vi "canmotor.vi"() -> (0 "x < y?":bool, 1 "两路电机速度":string, 2 "J45电机":dbl, 3 "J67电机":dbl)   [LabVIEW 2020]
uses:
  ControlCAN For LabVIEW8.6/ControlCAN.llb/VCI_CAN_OBJ.ctl
  ControlCAN For LabVIEW8.6/ControlCAN.llb/DevType.ctl
  ControlCAN For LabVIEW8.6/ControlCAN.llb/VCI_INIT_CONFIG.ctl
  ControlCAN For LabVIEW8.6/ControlCAN.llb/InitFlag.ctl
  ControlCAN For LabVIEW8.6/ControlCAN.llb/Fliter.ctl
  ControlCAN For LabVIEW8.6/ControlCAN.llb/Mode.ctl
  ControlCAN For LabVIEW8.6/ControlCAN.lvlib
panel:
  out "十进制整型字符串 2":string
  out "十进制整型字符串":string
  out "输出结果－电子表格字符串（'\\'代码显示） 2":string
  out "电机和":dbl
  out "Recieve 2":T1[](array[typedef])
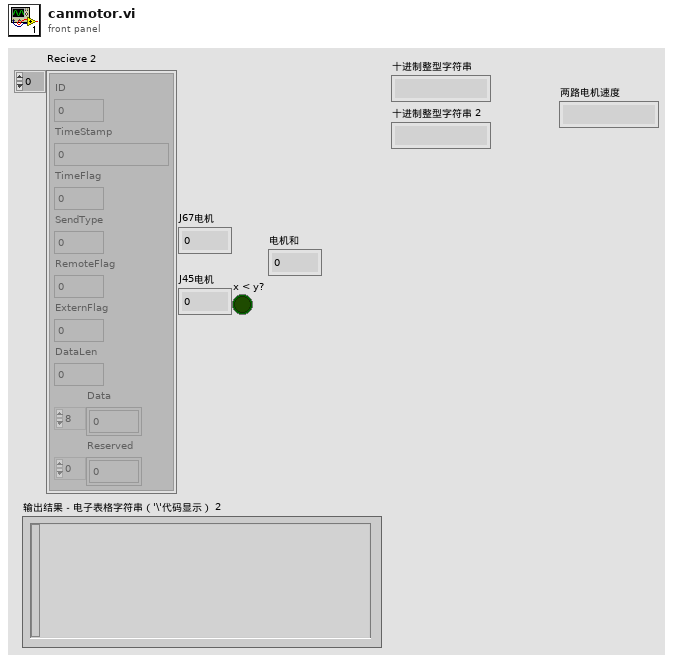
[diagram p1: front panel]
types:
  T1 = typedef "ControlCAN.lvlib/VCI_CAN_OBJ.ctl" = cluster{"ID":u32, "TimeStamp":u32, "TimeFlag":u8, "SendType":u8, "RemoteFlag":u8, "ExternFlag":u8, "DataLen":u8, "Data":u8[], "Reserved":u8[]}
  T2 = typedef "ControlCAN.lvlib/VCI_INIT_CONFIG.ctl" = cluster{"AccCode":u32, "AccMask":u32, "InitFlag":T3, "Fliter":T4, "Timing0":u8, "Timing1":u8, "Mode":T5}
  T3 = typedef "ControlCAN.lvlib/InitFlag.ctl" = u32
  T4 = typedef "ControlCAN.lvlib/Fliter.ctl" = u8
  T5 = typedef "ControlCAN.lvlib/Mode.ctl" = u8
  T6 = typedef "ControlCAN.lvlib/DevType.ctl" = u32
  T7 = cluster{"Recieve 2[0]":T1, "Recieve 2[1]":T1, "Recieve 2[2]":T1, "Recieve 2[3]":T1, "Recieve 2[4]":T1, "Recieve 2[5]":T1, "Recieve 2[6]":T1, "Recieve 2[7]":T1, "Recieve 2[8]":T1}
  T8 = cluster{"Data[0]":u8, "Data[1]":u8, "Data[2]":u8, "Data[3]":u8, "Data[4]":u8, "Data[5]":u8, "Data[6]":u8, "Data[7]":u8, "Data[8]":u8}
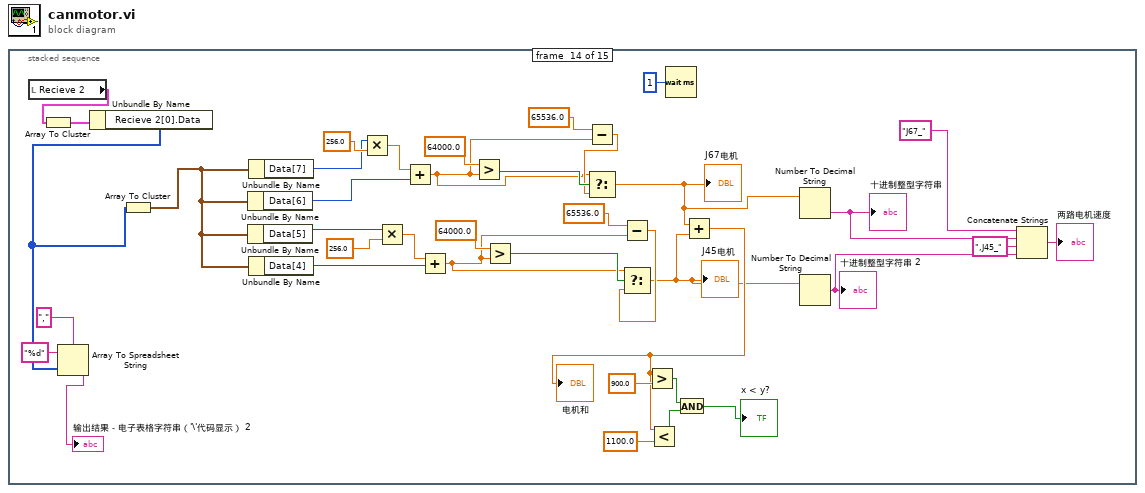
[diagram p0: block diagram]
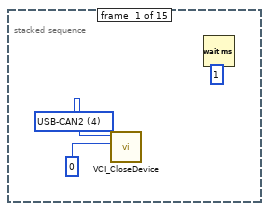
[diagram p2: hidden frame]
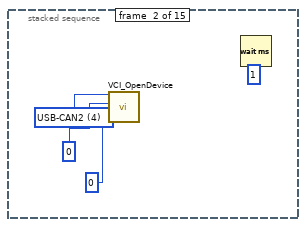
[diagram p3: hidden frame]
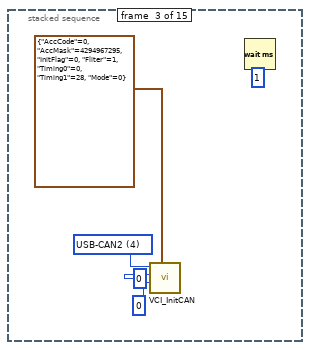
[diagram p4: hidden frame]
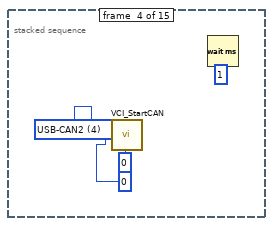
[diagram p5: hidden frame]
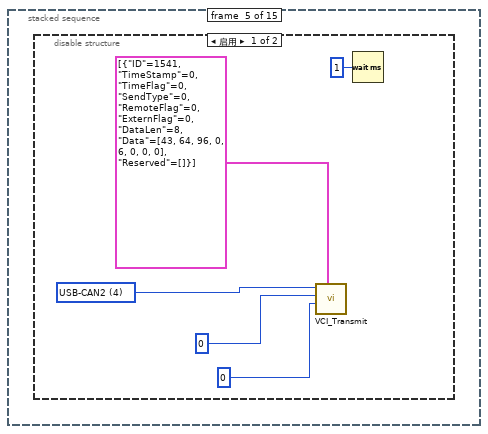
[diagram p6: hidden frame]
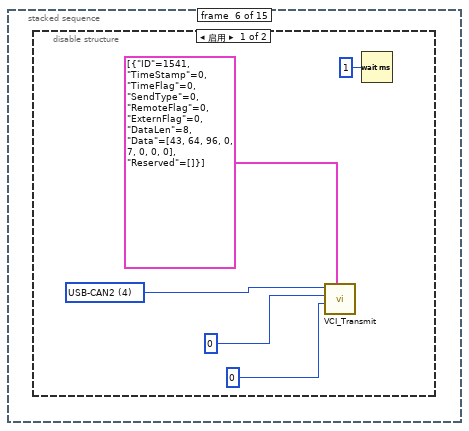
[diagram p8: hidden frame]
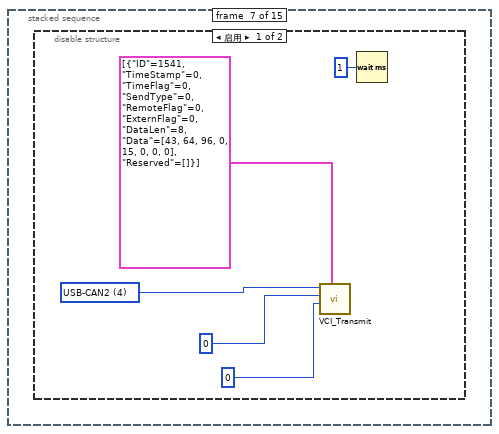
[diagram p10: hidden frame]
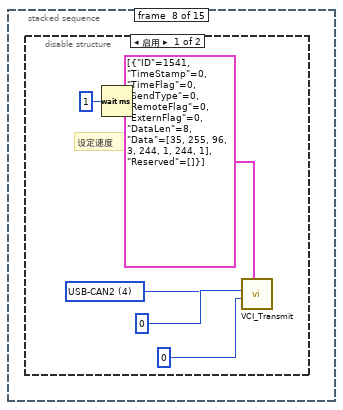
[diagram p12: hidden frame]
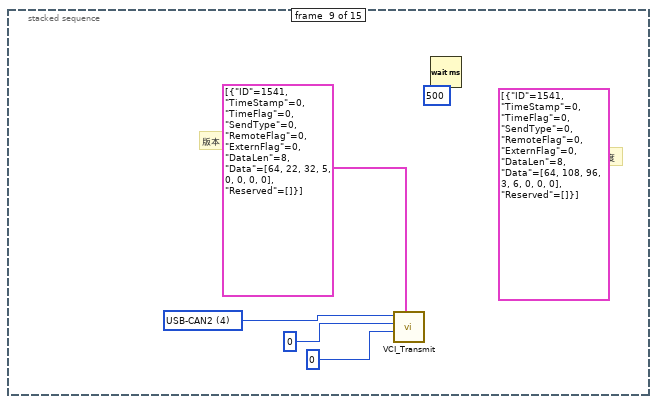
[diagram p14: hidden frame]
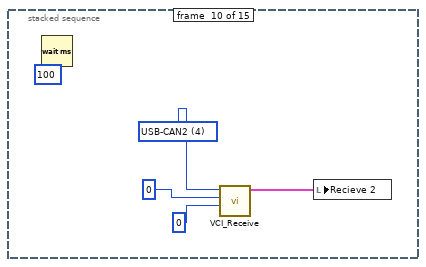
[diagram p15: hidden frame]
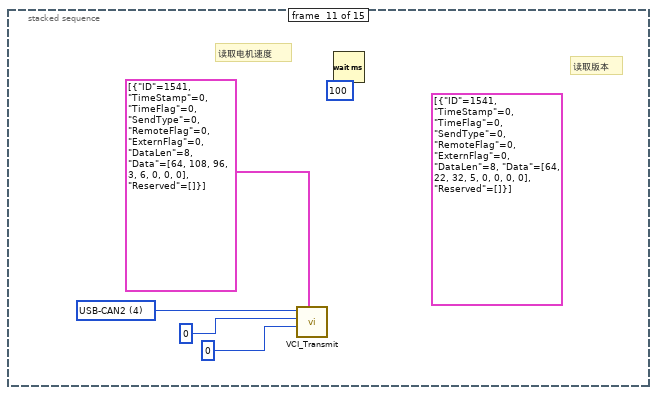
[diagram p16: hidden frame]
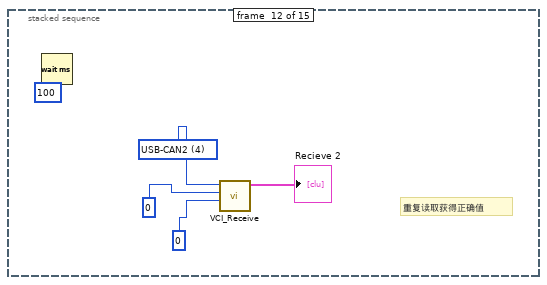
[diagram p17: hidden frame]
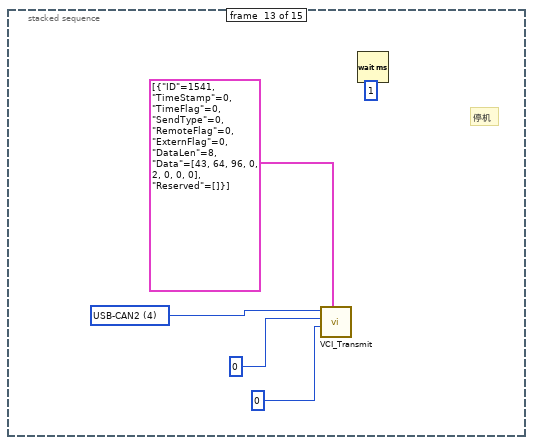
[diagram p18: hidden frame]
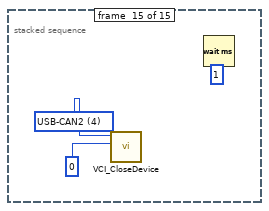
[diagram p19: hidden frame]
diagram:
  n1 = stacked-sequence {
    frame #0 {
      w3 = T6 4 items=["USB-CAN"=3, "USB-CAN2"=4] ("DevType")
      n2 = call "VCI_CloseDevice.vi"("DevIndex"=u32 0, "DevType"=w3) -> ()  [unwired: 8 in, 2 out]
      n3 = Wait (ms)(milliseconds to wait=u32 1 ("等待时间（毫秒）")) -> ()  [unwired: 1 out]
    }
    frame #1 {
      w5 = T6 4 items=["USB-CAN"=3, "USB-CAN2"=4] ("DevType")
      n4 = call "VCI_OpenDevice.vi"("Reserved"=u32 0, "DevIndex"=u32 0, "DevType"=w5) -> ()  [unwired: 1 in, 8 out]
      n5 = Wait (ms)(milliseconds to wait=u32 1 ("等待时间（毫秒）")) -> ()  [unwired: 1 out]
    }
    frame #2 {
      w9 = T6 4 items=["USB-CAN"=3, "USB-CAN2"=4] ("DevType")
      n6 = call "VCI_InitCAN.vi"("VCI_INIT_CONFIG"=T2 {"AccCode"=0, "AccMask"=4294967295, "InitFlag"=0, "Fliter"=1, "Timing0"=0, "Timing1"=28, "Mode"=0}, "CANIndex"=u32 0, "DevIndex"=u32 0, "DevType"=w9) -> ()  [unwired: 6 in, 2 out]
      n7 = Wait (ms)(milliseconds to wait=u32 1 ("等待时间（毫秒）")) -> ()  [unwired: 1 out]
    }
    frame #3 {
      w14 = T6 4 items=["USB-CAN"=3, "USB-CAN2"=4] ("DevType")
      n8 = call "VCI_StartCAN.vi"("CANIndex"=u32 0, "DevIndex"=u32 0, "DevType"=w14) -> ()  [unwired: 7 in, 2 out]
      n9 = Wait (ms)(milliseconds to wait=u32 1 ("等待时间（毫秒）")) -> ()  [unwired: 1 out]
    }
    frame #4 {
      n10 = disable-structure shown="启用" {
        frame Enabled {
          w18 = T6 4 items=["USB-CAN"=3, "USB-CAN2"=4] ("DevType")
          n11 = call "VCI_Transmit.vi"("Buffer"=T1[] [{"ID"=1541, "TimeStamp"=0, "TimeFlag"=0, "SendType"=0, "RemoteFlag"=0, "ExternFlag"=0, "DataLen"=8, "Data"=[43, 64, 96, 0, 6, 0, 0, 0], "Reserved"=[]}], "CANIndex"=u32 0, "DevIndex"=u32 0, "DevType"=w18) -> ()  [unwired: 6 in, 2 out]
          n12 = Wait (ms)(milliseconds to wait=u32 1 ("等待时间（毫秒）")) -> ()  [unwired: 1 out]
        }
        frame Disabled {
        }
      }
    }
    frame #5 {
      n13 = disable-structure shown="启用" {
        frame Enabled {
          w23 = T6 4 items=["USB-CAN"=3, "USB-CAN2"=4] ("DevType")
          n14 = call "VCI_Transmit.vi"("Buffer"=T1[] [{"ID"=1541, "TimeStamp"=0, "TimeFlag"=0, "SendType"=0, "RemoteFlag"=0, "ExternFlag"=0, "DataLen"=8, "Data"=[43, 64, 96, 0, 7, 0, 0, 0], "Reserved"=[]}], "CANIndex"=u32 0, "DevIndex"=u32 0, "DevType"=w23) -> ()  [unwired: 6 in, 2 out]
          n15 = Wait (ms)(milliseconds to wait=u32 1 ("等待时间（毫秒）")) -> ()  [unwired: 1 out]
        }
        frame Disabled {
        }
      }
    }
    frame #6 {
      n16 = disable-structure shown="启用" {
        frame Enabled {
          w28 = T6 4 items=["USB-CAN"=3, "USB-CAN2"=4] ("DevType")
          n17 = call "VCI_Transmit.vi"("Buffer"=T1[] [{"ID"=1541, "TimeStamp"=0, "TimeFlag"=0, "SendType"=0, "RemoteFlag"=0, "ExternFlag"=0, "DataLen"=8, "Data"=[43, 64, 96, 0, 15, 0, 0, 0], "Reserved"=[]}], "CANIndex"=u32 0, "DevIndex"=u32 0, "DevType"=w28) -> ()  [unwired: 6 in, 2 out]
          n18 = Wait (ms)(milliseconds to wait=u32 1 ("等待时间（毫秒）")) -> ()  [unwired: 1 out]
        }
        frame Disabled {
        }
      }
    }
    frame #7 {
      n19 = disable-structure shown="启用" {
        frame Enabled {
          w33 = T6 4 items=["USB-CAN"=3, "USB-CAN2"=4] ("DevType")
          # "设定速度"
          n20 = Wait (ms)(milliseconds to wait=u32 1 ("等待时间（毫秒）")) -> ()  [unwired: 1 out]
          n21 = call "VCI_Transmit.vi"("Buffer"=T1[] [{"ID"=1541, "TimeStamp"=0, "TimeFlag"=0, "SendType"=0, "RemoteFlag"=0, "ExternFlag"=0, "DataLen"=8, "Data"=[35, 255, 96, 3, 244, 1, 244, 1], "Reserved"=[]}], "CANIndex"=u32 0, "DevIndex"=u32 0, "DevType"=w33) -> ()  [unwired: 6 in, 2 out]
        }
        frame Disabled {
        }
      }
    }
    frame #8 {
      (unwired) T1[] [{"ID"=1541, "TimeStamp"=0, "TimeFlag"=0, "SendType"=0, "RemoteFlag"=0, "ExternFlag"=0, "DataLen"=8, "Data"=[64, 108, 96, 3, 6, 0, 0, 0], "Reserved"=[]}] ("Buffer")
      w39 = T6 4 items=["USB-CAN"=3, "USB-CAN2"=4] ("DevType")
      # "速度"
      # "版本"
      n22 = call "VCI_Transmit.vi"("Buffer"=T1[] [{"ID"=1541, "TimeStamp"=0, "TimeFlag"=0, "SendType"=0, "RemoteFlag"=0, "ExternFlag"=0, "DataLen"=8, "Data"=[64, 22, 32, 5, 0, 0, 0, 0], "Reserved"=[]}], "CANIndex"=u32 0, "DevIndex"=u32 0, "DevType"=w39) -> ()  [unwired: 6 in, 2 out]
      n23 = Wait (ms)(milliseconds to wait=u32 500 ("等待时间（毫秒）")) -> ()  [unwired: 1 out]
    }
    frame #9 {
      w46 = T6 4 items=["USB-CAN"=3, "USB-CAN2"=4] ("DevType")
      n24 = Wait (ms)(milliseconds to wait=u32 100 ("等待时间（毫秒）")) -> ()  [unwired: 1 out]
      n25 = call "VCI_Receive.vi"("CANIndex"=u32 0, "DevIndex"=u32 0, "DevType"=w46) -> ("Recieve"=w42:T1[])  [unwired: 3 in, 5 out]
      n26 = local write "Recieve 2"(w42) -> ()
    }
    frame #10 {
      (unwired) T1[] [{"ID"=1541, "TimeStamp"=0, "TimeFlag"=0, "SendType"=0, "RemoteFlag"=0, "ExternFlag"=0, "DataLen"=8, "Data"=[64, 22, 32, 5, 0, 0, 0, 0], "Reserved"=[]}] ("Buffer")
      w49 = T6 4 items=["USB-CAN"=3, "USB-CAN2"=4] ("DevType")
      # "读取版本"
      # "读取电机速度"
      n27 = call "VCI_Transmit.vi"("Buffer"=T1[] [{"ID"=1541, "TimeStamp"=0, "TimeFlag"=0, "SendType"=0, "RemoteFlag"=0, "ExternFlag"=0, "DataLen"=8, "Data"=[64, 108, 96, 3, 6, 0, 0, 0], "Reserved"=[]}], "CANIndex"=u32 0, "DevIndex"=u32 0, "DevType"=w49) -> ()  [unwired: 6 in, 2 out]
      n28 = Wait (ms)(milliseconds to wait=u32 100 ("等待时间（毫秒）")) -> ()  [unwired: 1 out]
    }
    frame #11 {
      w56 = T6 4 items=["USB-CAN"=3, "USB-CAN2"=4] ("DevType")
      # "重复读取获得正确值"
      n29 = Wait (ms)(milliseconds to wait=u32 100 ("等待时间（毫秒）")) -> ()  [unwired: 1 out]
      n30 = call "VCI_Receive.vi"("CANIndex"=u32 0, "DevIndex"=u32 0, "DevType"=w56) -> ("Recieve"=→"Recieve 2":T1[])  [unwired: 3 in, 5 out]
    }
    frame #12 {
      w58 = T6 4 items=["USB-CAN"=3, "USB-CAN2"=4] ("DevType")
      # "停机"
      n31 = call "VCI_Transmit.vi"("Buffer"=T1[] [{"ID"=1541, "TimeStamp"=0, "TimeFlag"=0, "SendType"=0, "RemoteFlag"=0, "ExternFlag"=0, "DataLen"=8, "Data"=[43, 64, 96, 0, 2, 0, 0, 0], "Reserved"=[]}], "CANIndex"=u32 0, "DevIndex"=u32 0, "DevType"=w58) -> ()  [unwired: 6 in, 2 out]
      n32 = Wait (ms)(milliseconds to wait=u32 1 ("等待时间（毫秒）")) -> ()  [unwired: 1 out]
    }
    frame #13 {
      n33 = local read "Recieve 2"() -> (w99:T1[])
      n34 = Array To Cluster(array=w99) -> (cluster=w93:T7)
      n35 = Unbundle By Name(w93) -> ("Recieve 2[0].Data"=w91:u8[])
      n36 = Array To Spreadsheet String(delimiter (Tab)="," ("分隔符(Tab)"), array=w91, 3:"%d" ("格式字符串")) -> (spreadsheet string=→"输出结果－电子表格字符串（'\\'代码显示） 2":string)
      n37 = Array To Cluster(array=w91) -> (cluster=w92:T8)
      n38 = Unbundle By Name(w92) -> ("Data[6]"=w90:u8)
      n39 = Unbundle By Name(w92) -> ("Data[5]"=w86:u8)
      n40 = Unbundle By Name(w92) -> ("Data[7]"=w94:u8)
      n41 = Unbundle By Name(w92) -> ("Data[4]"=w85:u8)
      n42 = Multiply(x=w94, y=256.0) -> (x*y=w89:dbl)
      n43 = Multiply(x=w86, y=256.0) -> (x*y=w88:dbl)
      n44 = Add(x=w89, y=w90) -> (x+y=w79:dbl)
      n45 = Add(x=w88, y=w85) -> (x+y=w75:dbl)
      n46 = Greater?(x=64000.0, y=w79) -> (0:w82:bool)
      n47 = Greater?(x=64000.0, y=w75) -> (0:w76:bool)
      n48 = Subtract(x=65536.0, y=w79) -> (x-y=w80:dbl)
      n49 = Select(t=w79, s=w82, f=w80) -> (s? t:f=w68:dbl)
      "J67电机" <- w68
      n50 = Subtract(x=65536.0, y=w75) -> (x-y=w78:dbl)
      n51 = Select(t=w75, s=w76, f=w78) -> (s? t:f=w67:dbl)
      "J45电机" <- w67
      n52 = Wait (ms)(milliseconds to wait=u32 1 ("等待时间（毫秒）")) -> ()  [unwired: 1 out]
      n53 = Add(x=w68, y=w67) -> (x+y=w73:dbl)
      "电机和" <- w73
      n54 = Greater?(x=w73, y=900.0) -> (0:w70:bool)
      n55 = Less?(x=w73, y=1100.0) -> (x < y?=w71:bool)
      n56 = And(x=w70, y=w71) -> (x .and. y?=→"x < y?":bool)
      n57 = Number To Decimal String(number=w68) -> (decimal integer string=w65:string)  [unwired: 1 in]
      "十进制整型字符串" <- w65
      n58 = Number To Decimal String(number=w67) -> (decimal integer string=w63:string)  [unwired: 1 in]
      "十进制整型字符串 2" <- w63
      n59 = Concatenate Strings("J67_" ("字符串"), w65, ",J45_" ("字符串"), w63) -> (→"两路电机速度":string)
    }
    frame #14 {
      w103 = T6 4 items=["USB-CAN"=3, "USB-CAN2"=4] ("DevType")
      n60 = call "VCI_CloseDevice.vi"("DevIndex"=u32 0, "DevType"=w103) -> ()  [unwired: 8 in, 2 out]
      n61 = Wait (ms)(milliseconds to wait=u32 1 ("等待时间（毫秒）")) -> ()  [unwired: 1 out]
    }
  }
